vi "Добавить точку на рисунок (SubVI).vi"(0 "in picture":picture, 1 "dot х":u16 step=1, 2 "dot y":u16 step=1, 3 "thickness":u16 step=1, 4 "цвет":u32(colorbox), 5 "error in":errorcluster) -> (14 "out picture":picture, 19 "error out":errorcluster)   [LabVIEW 2013]
panel:
  in  "Style":T1(ring)
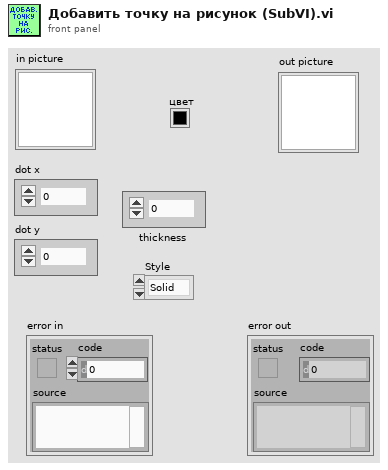
[diagram p1: front panel]
types:
  T1 = enum32{"Solid", "Dash", "Dot", "DashDot", "DashDotDot"}
  T2 = cluster{"thickness":u16, "Style":enum32{"Solid", "Dash", "Dot", "DashDot", "DashDotDot"}}
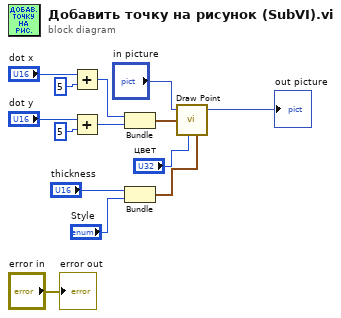
[diagram p0: block diagram]
diagram:
  n1 = Add(x="dot х", y=u16 5) -> (x+y=w1:u16)
  n2 = Add(x="dot y", y=u16 5) -> (x+y=w2:u16)
  n3 = Bundle(w1, w2) -> (w10:cluster{u16, u16})  [unwired: 1 in]
  n4 = Bundle("thickness"="thickness", "Style"="Style") -> (w13:T2)  [unwired: 1 in]
  n5 = call <vilib>:"Draw Point.vi"("picture"="in picture", "point(x,y)"=w10, "color(black)"="цвет", "pen"=w13) -> ("new picture"=→"out picture":picture)  [unwired: 5 in]
  "error out" <- "error in"
